vi "gotoxy.vi"(8 "error in":T1, 10 "yPos":sgl format="%#_g nm", 11 "xPos":sgl format="%#_g nm") -> (0 "error out":T1)   [LabVIEW 2016]
doc: "By the help of this VI the scanner can be moved to a specific xy-Position (input values)."
uses:
  Controls/Error_Out.ctl
  Files_ASC500/DLL/ASC500_RemoteControlV27.dll
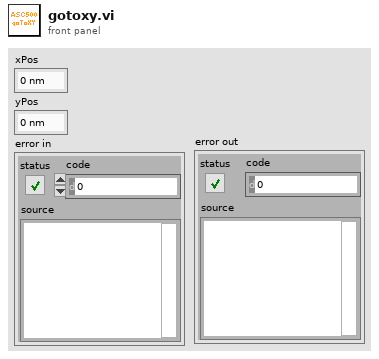
[diagram p1: front panel]
types:
  T1 = typedef "Error_Out.ctl" = errorcluster
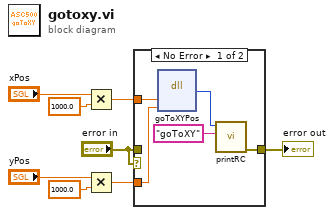
[diagram p0: block diagram]
diagram:
  n1 = Multiply(x="xPos", y=sgl 1000.0) -> (x*y=w4:sgl)
  n2 = Multiply(x="yPos", y=sgl 1000.0) -> (x*y=w2:sgl)
  n3 = case shown="No Error" "error in" {
    tunnel: "error in" -> [_ w14]
    tunnel: [w9 w14] -> w7
    tunnel: w4 -> [w13 _]
    tunnel: w2 -> [w12 _]
    frame No Error {
      n4 = dll-call lib="G:/SCMOperations/Share/ELE/Produkt Information/ASC500/04 Remote Control/01 released remote control versions/V27/ASC500 Remote Control Release Candidate 0.2.1 2019.09.04/Files_ASC500/DLL/ASC500_RemoteControlV27.dll" fn="goToXYPos"("xPos"=w13, "yPos"=w12) -> ("return code"=w11:i32)  [unwired: 5 in, 2 out]
      n5 = call "printRC.vi"("additional information"="goToXY", "RC"=w11) -> ("error out"=w9:T1)  [unwired: 9 in]
    }
    frame Error {
    }
  }
  "error out" <- w7
